vi "Calculate Part Average.vi"(11 "Avg Array":dbl[][](array[numeric])) -> (3 "Parts Averages":dbl)   [LabVIEW 2018, in "GRR Core.lvclass"]
uses:
  GRR Core.lvclass
  <vilib>/Analysis/baseanly.llb/Mean (DBL).vi
  <vilib>/Analysis/NI_AALBase.lvlib
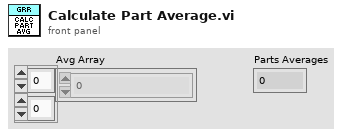
[diagram p1: front panel]
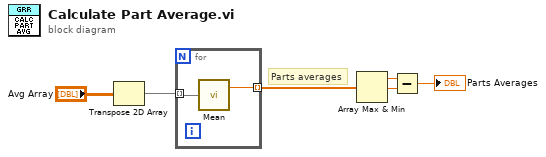
[diagram p0: block diagram]
diagram:
  # "Parts averages"
  n1 = Transpose 2D Array(2D array="Avg Array") -> (transposed array=w2:dbl[][])
  n2 = for {
    tunnel: w2 -> [w8] mode=indexing
    tunnel: [w7] -> w6 mode=indexing
    n3 = call-poly <vilib>:"Mean.vi"("X"=w8) -> ("mean"=w7:dbl)  [unwired: 1 out]
  }
  n4 = Array Max & Min(array=w6) -> (max value=w5:dbl, min value=w4:dbl)  [unwired: 2 out]
  n5 = Subtract(x=w5, y=w4) -> (x-y=→"Parts Averages":dbl)
